vi "Dequeue Message.vi"(8 "error in (no error)":errorcluster, 11 "PID Loop in":refnum<class "PID Loop.lvclass">) -> (0 "error out":errorcluster, 1 "Data":variant, 2 "Message":T1, 3 "PID Loop out":refnum<class "PID Loop.lvclass">)   [LabVIEW 2024, in "PID Loop.lvlib" / "PID Loop.lvclass"]
uses:
  PID Loop.lvclass
  PID Loop.lvclass/PID Loop.ctl
  Messages.ctl
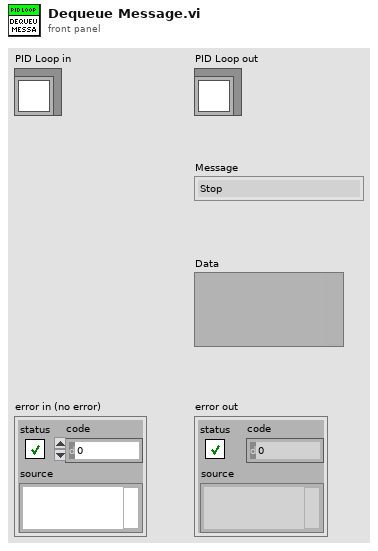
[diagram p1: front panel]
types:
  T1 = typedef "PID Loop.lvlib/PID Loop.lvclass/Messages.ctl" = enum16{"Stop", "Start", "Exit", "Poll"}
  T2 = typedef "PID Loop.lvlib/PID Loop.lvclass/Message.ctl" = cluster{"Message":T1, "Data":variant}
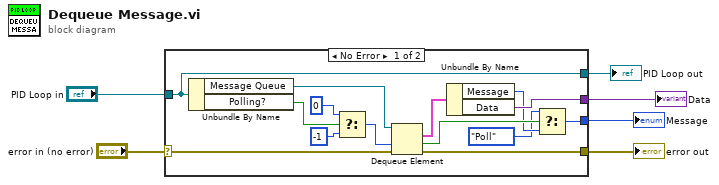
[diagram p0: block diagram]
diagram:
  n1 = case shown="No Error" "error in (no error)" {
    selector: "error in (no error)" -> [w18 w22]
    tunnel: [w17 w22] -> w5
    tunnel: [w20 w21] -> w3
    tunnel: "PID Loop in" -> [w20 w21]
    tunnel: [w8 _] -> w2
    tunnel: [w10 _] -> w1
    frame No Error {
      n2 = Unbundle By Name(w20) -> ("Message Queue"=w19:refnum<queue>, "Polling?"=w16:bool)
      n3 = Select(t=0, s=w16, f=-1) -> (s? t:f=w12:i32)
      n4 = Dequeue Element(queue=w19, timeout in ms (-1)=w12, error in (no error)=w18) -> (element=w11:T2, timed out?=w15:bool, error out=w17:errorcluster)  [unwired: 1 out]
      n5 = Unbundle By Name(w11) -> ("Message"=w9:T1, "Data"=w10:variant)
      n6 = Select(t=Messages."Poll" ("Message"), s=w15, f=w9) -> (s? t:f=w8:T1)
    }
    frame Error {
    }
  }
  "error out" <- w5
  "PID Loop out" <- w3
  "Message" <- w2
  "Data" <- w1
